vi "Part 2.vi"(11 "Input":string) -> (3 "Output":dbl format="%#.6f")   [LabVIEW 2021]
uses:
  <vilib>/Analysis/NI_AALBase.lvlib
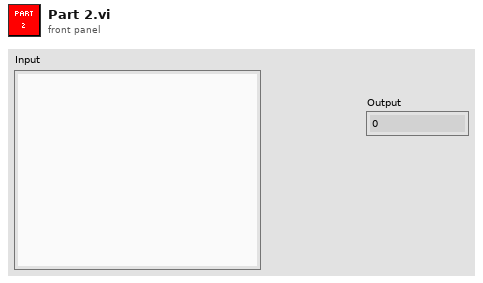
[diagram p1: front panel]
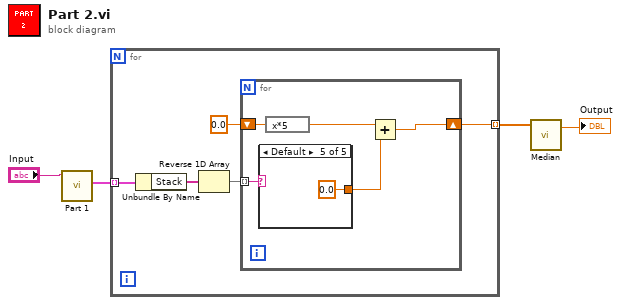
[diagram p0: block diagram]
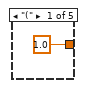
[diagram p2: hidden frame]
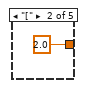
[diagram p3: hidden frame]
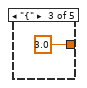
[diagram p4: hidden frame]
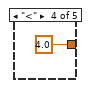
[diagram p5: hidden frame]
diagram:
  n1 = call "Part 1.vi"("Input"="Input") -> ("Incomplete Stacks"=w3:cluster{"Stack":string[]}[])  [unwired: 9 in, 1 out]
  n2 = for {
    tunnel: w3 -> [w9] mode=indexing
    tunnel: [w5] -> w1 mode=indexing
    n3 = Unbundle By Name(w9) -> ("Stack"=w8:string[])
    n4 = Reverse 1D Array(array=w8) -> (reversed array=w7:string[])
    n5 = for {
      tunnel: w7 -> [w14] mode=indexing
      shift-right: [w11] -> w5
      shift-left: 0.0 -> [w12]
      n6 = case shown="Default" w14 {
        tunnel: [1.0 2.0 3.0 4.0 0.0] -> w10
        frame "(" {
        }
        frame "[" {
        }
        frame "{" {
        }
        frame "<" {
        }
        frame Default {
        }
      }
      n7 = expression code="x*5"(w12) -> (w13:dbl)
      n8 = Add(x=w13, y=w10) -> (x+y=w11:dbl)
    }
  }
  n9 = call <vilib>:"Median.vi"("X"=w1) -> ("median"=→"Output":dbl)  [unwired: 1 out]
